vi "RampVoltage.vi"(0 "VISA resource name":refnum<visa-resource-name>, 1 "Delay (s)":dbl=0.2, 5 "Current voltage (V)":dbl, 7 "Target voltage (V)":dbl, 9 "Compliance Current (A)":dbl=0.1, 11 "error in (no error)":errorcluster, 12 "Step size (V)":dbl=50.0) -> (4 "VISA resource name out":refnum<visa-resource-name>, 6 "Current voltage out (V)":dbl, 15 "error out":errorcluster)   [LabVIEW 2015]
uses:
  Program Files (x86)/National Instruments/LabVIEW 2016/instr.lib/Keithley 24XX/Keithley 24XX.lvlib
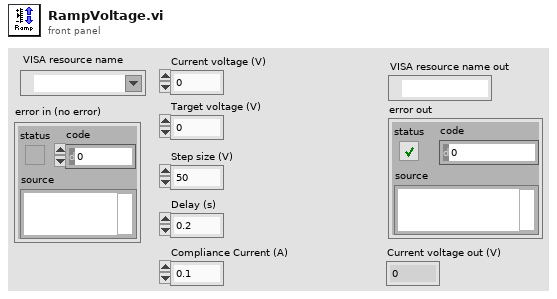
[diagram p1: front panel]
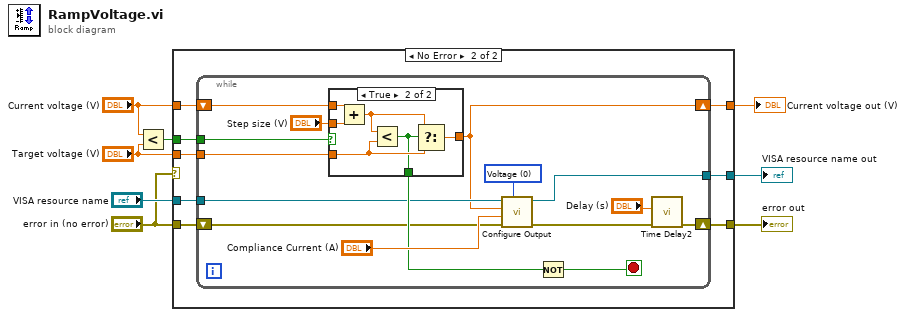
[diagram p0: block diagram]
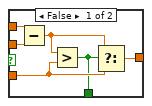
[diagram p3: hidden frame]
diagram:
  n1 = Less?(x="Current voltage (V)", y="Target voltage (V)") -> (x < y?=w6:bool)
  n2 = case shown="No Error" "error in (no error)" {
    tunnel: "error in (no error)" -> [w10 w19]
    tunnel: "Target voltage (V)" -> [_ w18]
    tunnel: "Current voltage (V)" -> [w11 w17]
    tunnel: w6 -> [_ w16]
    tunnel: "VISA resource name" -> [w9 w15]
    tunnel: [w9 w14] -> w4
    tunnel: [w10 w13] -> w3
    tunnel: [w11 w12] -> w2
    frame Error {
    }
    frame No Error {
      n3 = while {
        shift-right: [w33] -> w13
        shift-left: w19 -> [w22]
        shift-right: [w21] -> w12
        shift-left: w17 -> [w29]
        tunnel: w18 -> [w31]
        tunnel: w16 -> [w32]
        tunnel: w15 -> [w23]
        tunnel: [w25] -> w14
        stop <- w20 stop-if-true
        w27 = u16 0 items=["Voltage", "Current"] ("Source Mode  (0: Voltage)")
        n4 = case shown="True" w32 {
          tunnel: w31 -> [w37 w43]
          tunnel: "Step size (V)" -> [w39 w45]
          tunnel: w29 -> [w40 w46]
          tunnel: [w36 w42] -> w21
          tunnel: [w35 w41] -> w24
          frame False {
            n5 = Subtract(x=w40, y=w39) -> (x-y=w38:dbl)
            n6 = Greater?(x=w38, y=w37) -> (0:w35:bool)
            n7 = Select(t=w38, s=w35, f=w37) -> (s? t:f=w36:dbl)
          }
          frame True {
            n8 = Add(x=w46, y=w45) -> (x+y=w44:dbl)
            n9 = Less?(x=w44, y=w43) -> (x < y?=w41:bool)
            n10 = Select(t=w44, s=w41, f=w43) -> (s? t:f=w42:dbl)
          }
        }
        n11 = call "Configure Output.vi"("Source Mode  (0: Voltage)"=w27, "error in (no error)"=w22, "Compliance  Level (0.1)"="Compliance Current (A)", "Output Level (0)"=w21, "VISA resource name"=w23) -> ("error out"=w26:errorcluster, "VISA resource name out"=w25:refnum<visa-resource-name>)  [unwired: 5 in]
        n12 = Not(x=w24) -> (.not. x?=w20:bool)
        n13 = call "Time Delay2"("error in (no error)"=w26, "Delay Time (s)"="Delay (s)") -> ("error out"=w33:errorcluster)  [unwired: 9 in]
      }
    }
  }
  "VISA resource name out" <- w4
  "error out" <- w3
  "Current voltage out (V)" <- w2
